vi "Update Status.vi"(8 "error in (no error)":errorcluster, 11 "Framework in":refnum<class "Framework.lvclass">) -> (0 "error out":errorcluster, 3 "Framework out":refnum<class "Framework.lvclass">)   [LabVIEW 2019, in "DSF Core.lvlib" / "Framework.lvclass"]
uses:
  Framework.lvclass
  Status/Status Data.ctl
  Framework.lvclass/Framework.ctl
  Status/Status Pointer.lvclass
  Plugin/Plugin.lvclass
  Performance/Performance.lvclass
  Framework Status/Framework Status.lvclass
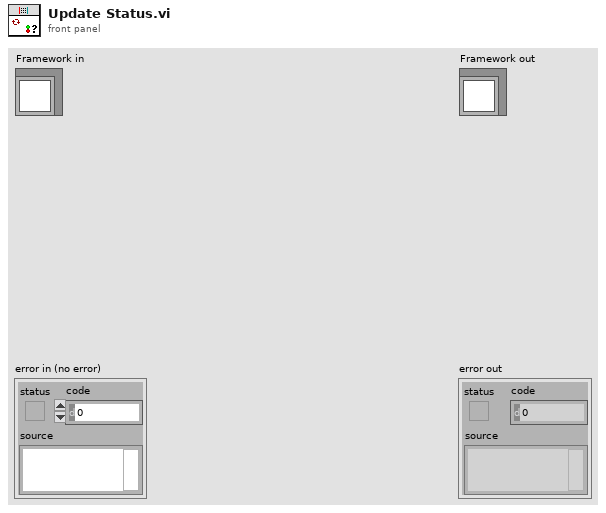
[diagram p1: front panel]
types:
  T1 = typedef "DSF Core.lvlib/Status Pointer.lvclass/Status Data.ctl" = cluster{"duration":u64, "period":u64, "iteration":u64, "late count":u64}
  T2 = typedef "DSF Core.lvlib/Timing Status Pointer.lvclass/Timing Status Data.ctl" = cluster{"rx start time":u32, "rx end time":u32, "tx start time":u32, "tx end time":u32, "cycle start time":u32, "cycle end time":u32, "prev start time":u32}
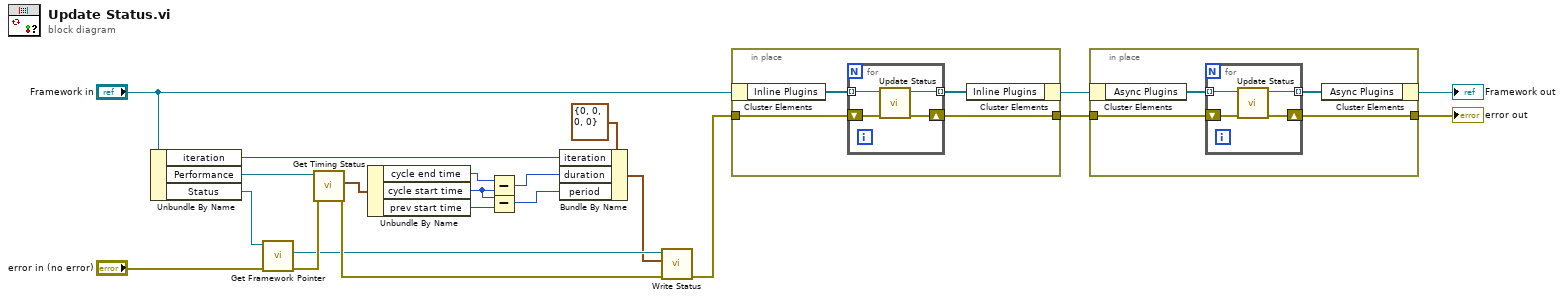
[diagram p0: block diagram]
diagram:
  n1 = Unbundle By Name("Framework in") -> ("iteration"=w21:u64, "Performance"=w11:refnum<class "Performance.lvclass">, "Status"=w13:refnum<class "Framework Status.lvclass">)
  n2 = call "Get Framework Pointer.vi"("error in (no error)"="error in (no error)", "Framework Status in"=w13) -> ("error out"=w10:errorcluster, "framework pointer"=w6:refnum<class "Status Pointer.lvclass">)  [unwired: 7 in, 1 out]
  n3 = call "Get Timing Status.vi"("error in (no error)"=w10, "Framework Performance in"=w11) -> ("error out"=w9:errorcluster, "timing status"=w8:T2)  [unwired: 7 in, 1 out]
  n4 = Unbundle By Name(w8) -> ("cycle end time"=w7:u32, "cycle start time"=w2:u32, "prev start time"=w3:u32)
  n5 = Subtract(x=w7, y=w2) -> (x-y=w5:u32)
  n6 = Subtract(x=w2, y=w3) -> (x-y=w1:u32)
  n7 = Bundle By Name(cluster=T1 {"duration"=0, "period"=0, "iteration"=0, "late count"=0} ("status"), "iteration"=w21, "duration"=w5, "period"=w1) -> (w4:T1)
  n8 = call "Write Status.vi"("error in (no error)"=w9, "status"=w4, "status pointer in"=w6) -> ("error out"=w20:errorcluster)  [unwired: 7 in, 1 out]
  n9 = in-place {
    in-place-border: [w23] -> w18
    in-place-border: w20 -> [w22]
    n10 = in-place-cluster #1("Framework in") -> ("Inline Plugins"=w25:refnum<class "Plugin.lvclass">[])
    n11 = for {
      tunnel: w25 -> [w29] mode=indexing
      tunnel: [w28] -> w24 mode=indexing
      shift-right: [w27] -> w23
      shift-left: w22 -> [w26]
      n12 = call "Update Status.vi"("error in (no error)"=w26, "Plugin in"=w29) -> ("error out"=w27:errorcluster, "Plugin out"=w28:refnum<class "Plugin.lvclass">)  [unwired: 8 in]
    }
    n13 = in-place-cluster #1("Inline Plugins"=w24) -> (w19:refnum<class "Framework.lvclass">)
  }
  n14 = in-place {
    in-place-border: [w31] -> w16
    in-place-border: w18 -> [w30]
    n15 = in-place-cluster #2(w19) -> ("Async Plugins"=w33:refnum<class "Plugin.lvclass">[])
    n16 = for {
      tunnel: w33 -> [w37] mode=indexing
      tunnel: [w36] -> w32 mode=indexing
      shift-right: [w35] -> w31
      shift-left: w30 -> [w34]
      n17 = call "Update Status.vi"("error in (no error)"=w34, "Plugin in"=w37) -> ("error out"=w35:errorcluster, "Plugin out"=w36:refnum<class "Plugin.lvclass">)  [unwired: 8 in]
    }
    n18 = in-place-cluster #2("Async Plugins"=w32) -> (→"Framework out":refnum<class "Framework.lvclass">)
  }
  "error out" <- w16
